vi "Generate PWM Signal Changing Frequency.vi"(5 "Frequency Min":dbl=1000.0 format="%.2f", 6 "Pulses per Revolution":i32=2000, 7 "Frequency Max":dbl=5000.0 format="%.2f", 8 "Duty Cycle":dbl=0.5 min=0.0 max=1.0 format="%#.2f", 9 "Ramp Down Duration":dbl=1.0, 10 "Constant Duration":dbl=1.0, 11 "Ramp Up Duration":dbl=1.0) -> (0 "Total Duration":dbl, 1 "Number of Samples":i32=1000, 2 "Frequency Duty Cycle Data":cluster{"duty cycle":dbl, "frequency":dbl}[](array[cluster]), 3 "Digital Waveform Graph":digitalwaveform(graph))   [LabVIEW 2017]
uses:
  <vilib>/Waveform/DTblOps.llb/DTbl Boolean Array to Digital.vi
panel:
  out "Waveform Graph":waveform(dbl)(graph)
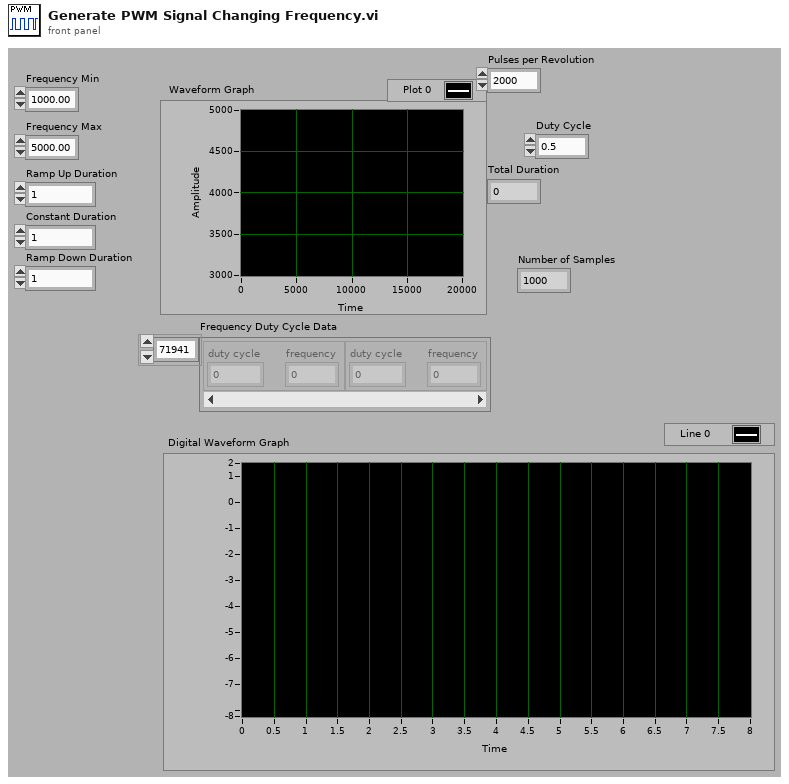
[diagram p1: front panel]
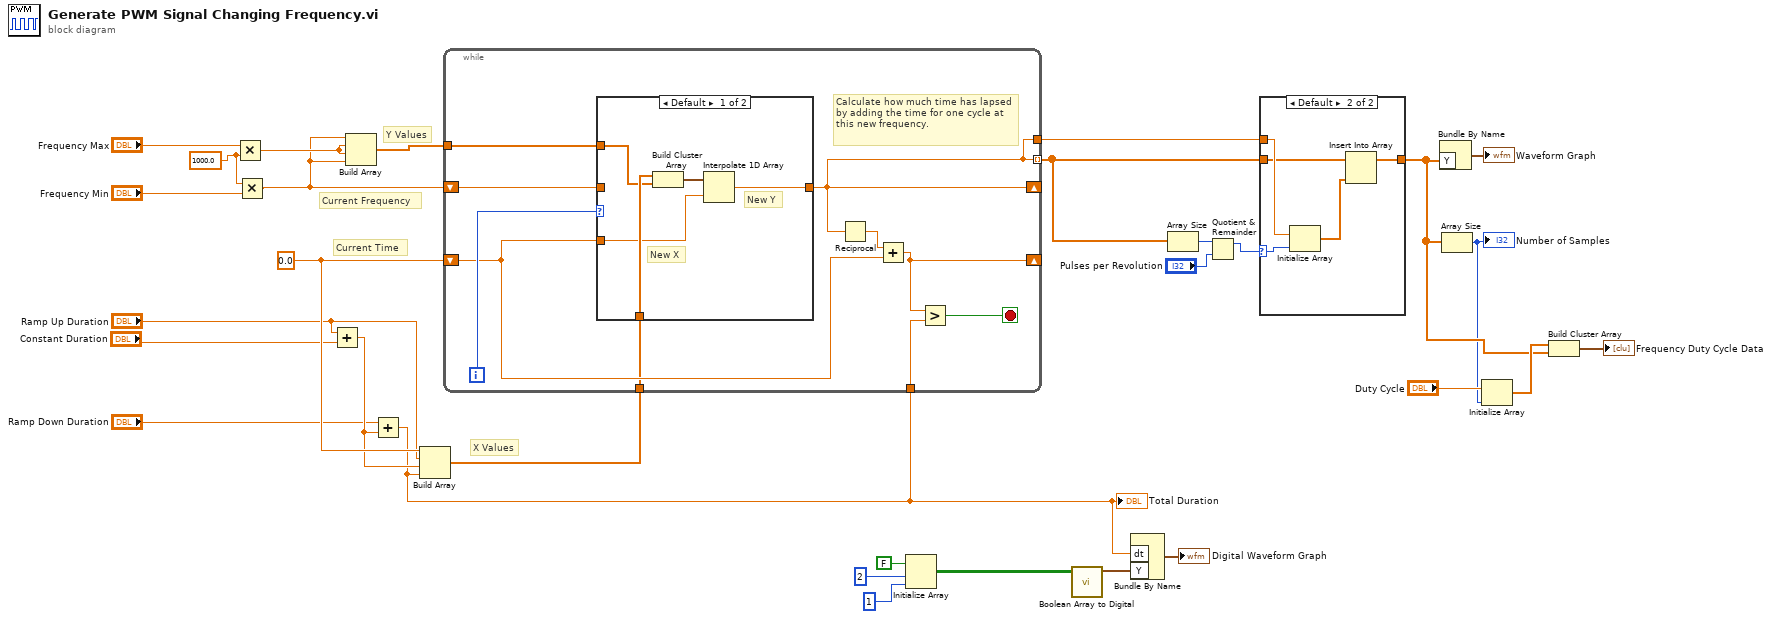
[diagram p0: block diagram]
diagram:
  w10 = 1000.0 ("y")
  w27 = 0.0 ("element")
  # "Current Frequency"
  # "Current Time"
  # "Y Values"
  # "X Values"
  n1 = Multiply(x="Frequency Max", y=w10) -> (x*y=w9:dbl)
  n2 = Multiply(x=w10, y="Frequency Min") -> (x*y=w8:dbl)
  n3 = Add(x="Ramp Up Duration", y="Constant Duration") -> (x+y=w22:dbl)
  n4 = Build Array(w8, w9, w9, w8) -> (w25:dbl[])
  n5 = Add(x="Ramp Down Duration", y=w22) -> (x+y=w2:dbl)
  "Total Duration" <- w2
  n6 = Build Array(w27, "Ramp Up Duration", w22, w2) -> (w26:dbl[])
  n7 = while {
    shift-right: [w34] -> _
    shift-left: w27 -> [w37]
    shift-right: [w31] -> _
    shift-left: w8 -> [w40]
    tunnel: w26 -> [w36]
    tunnel: w25 -> [w35]
    tunnel: w2 -> [w33]
    tunnel: [w31] -> w16 mode=indexing
    tunnel: [w31] -> w13
    i -> [w38]
    stop <- w32 stop-if-true
    # "Calculate how much time has lapsed by adding the time for one cycle at this new frequency."
    n8 = case shown="Default" w38 {
      tunnel: w40 -> [_ w46]
      tunnel: [w41 w46] -> w31
      tunnel: w37 -> [w42 _]
      tunnel: w36 -> [w45 _]
      tunnel: w35 -> [w44 _]
      frame Default {
        # "New Y"
        # "New X"
        n9 = Build Cluster Array(w45, w44) -> (w43:cluster{"Ramp Up Duration":dbl, dbl}[])
        n10 = Interpolate 1D Array(1:w42, 2:w43) -> (0:w41:dbl)
      }
      frame 0 {
        # "Start at minimum"
      }
    }
    n11 = Reciprocal(x=w31) -> (1/x=w39:dbl)
    n12 = Add(x=w39, y=w37) -> (x+y=w34:dbl)
    n13 = Greater?(x=w34, y=w33) -> (0:w32:bool)
  }
  n14 = Initialize Array(FALSE, 2 ("dimension size"), 1 ("dimension size")) -> (w4:bool[][])
  n15 = call-poly <vilib>:"Boolean Array to Digital.vi"("boolean array"=w4) -> ("digital data"=w7:digitaldata)  [unwired: 3 in, 7 out]
  n16 = Bundle By Name("dt"=w2, "Y"=w7) -> (→"Digital Waveform Graph":digitalwaveform)  [unwired: 1 in]
  n17 = Array Size(array=w16) -> (size(s)=w19:i32)
  n18 = Quotient & Remainder(x=w19, y="Pulses per Revolution") -> (x-y*floor(x/y)=w17:i32)  [unwired: 1 out]
  n19 = case shown="Default" w17 {
    selector: w17 -> [_ w52]
    tunnel: w16 -> [w47 w50]
    tunnel: [w47 w48] -> w15
    tunnel: w13 -> [_ w51]
    frame 0 {
    }
    frame Default {
      n20 = Initialize Array(w51, w52) -> (w49:dbl[])
      n21 = Insert Into Array(array=w50, new element=w49) -> (w48:dbl[])  [unwired: 1 in]
    }
  }
  n22 = Bundle By Name("Y"=w15) -> (→"Waveform Graph":waveform(dbl))  [unwired: 1 in]
  n23 = Array Size(array=w15) -> (size(s)=w14:i32)
  "Number of Samples" <- w14
  n24 = Initialize Array("Duty Cycle", w14) -> (w29:dbl[])
  n25 = Build Cluster Array(w29, w15) -> (→"Frequency Duty Cycle Data":cluster{"Duty Cycle":dbl, dbl}[])
